vi "interface-doan.vi"() -> ()   [LabVIEW 2015]
panel:
  in  "?":T1(tab)
  out "Complete!":bool
  in  "?":bool
  in  "?":bool
  out "Process":dbl(knob) scale=0.0..100.0
  in  "?":path
  in  "GATE-3 3":i32(listbox)
  out "Complete!":bool
  in  "?":bool
  in  "?":bool
  out "Process":dbl(knob) scale=0.0..100.0
  in  "?":path
  in  "GATE-2 2":i32(listbox)
  out "Complete!":bool
  in  "?":bool
  in  "?":bool
  out "Process":dbl(knob) scale=0.0..100.0
  in  "?":path
  in  "GATE-1":i32(listbox)
  out "3":bool
  out "2":bool
  out "1":bool
  in  "Value 2":dbl
  in  "Value 1":dbl
  in  "Calibration":dbl
  in  "ERROR":errorcluster
  in  "ERROR":errorcluster
  out "Processing Chart":dbl(graph)
  out "WEIGHT PASS":bool
  out "Measurement\nValue":dbl
  out "Calculated\nValue":dbl
  out "Frame rate":dbl
  in  "DATA":string
  out "FOUND-QR":bool
  out "?":T2(plugin-control)
  # "GATE OUT"
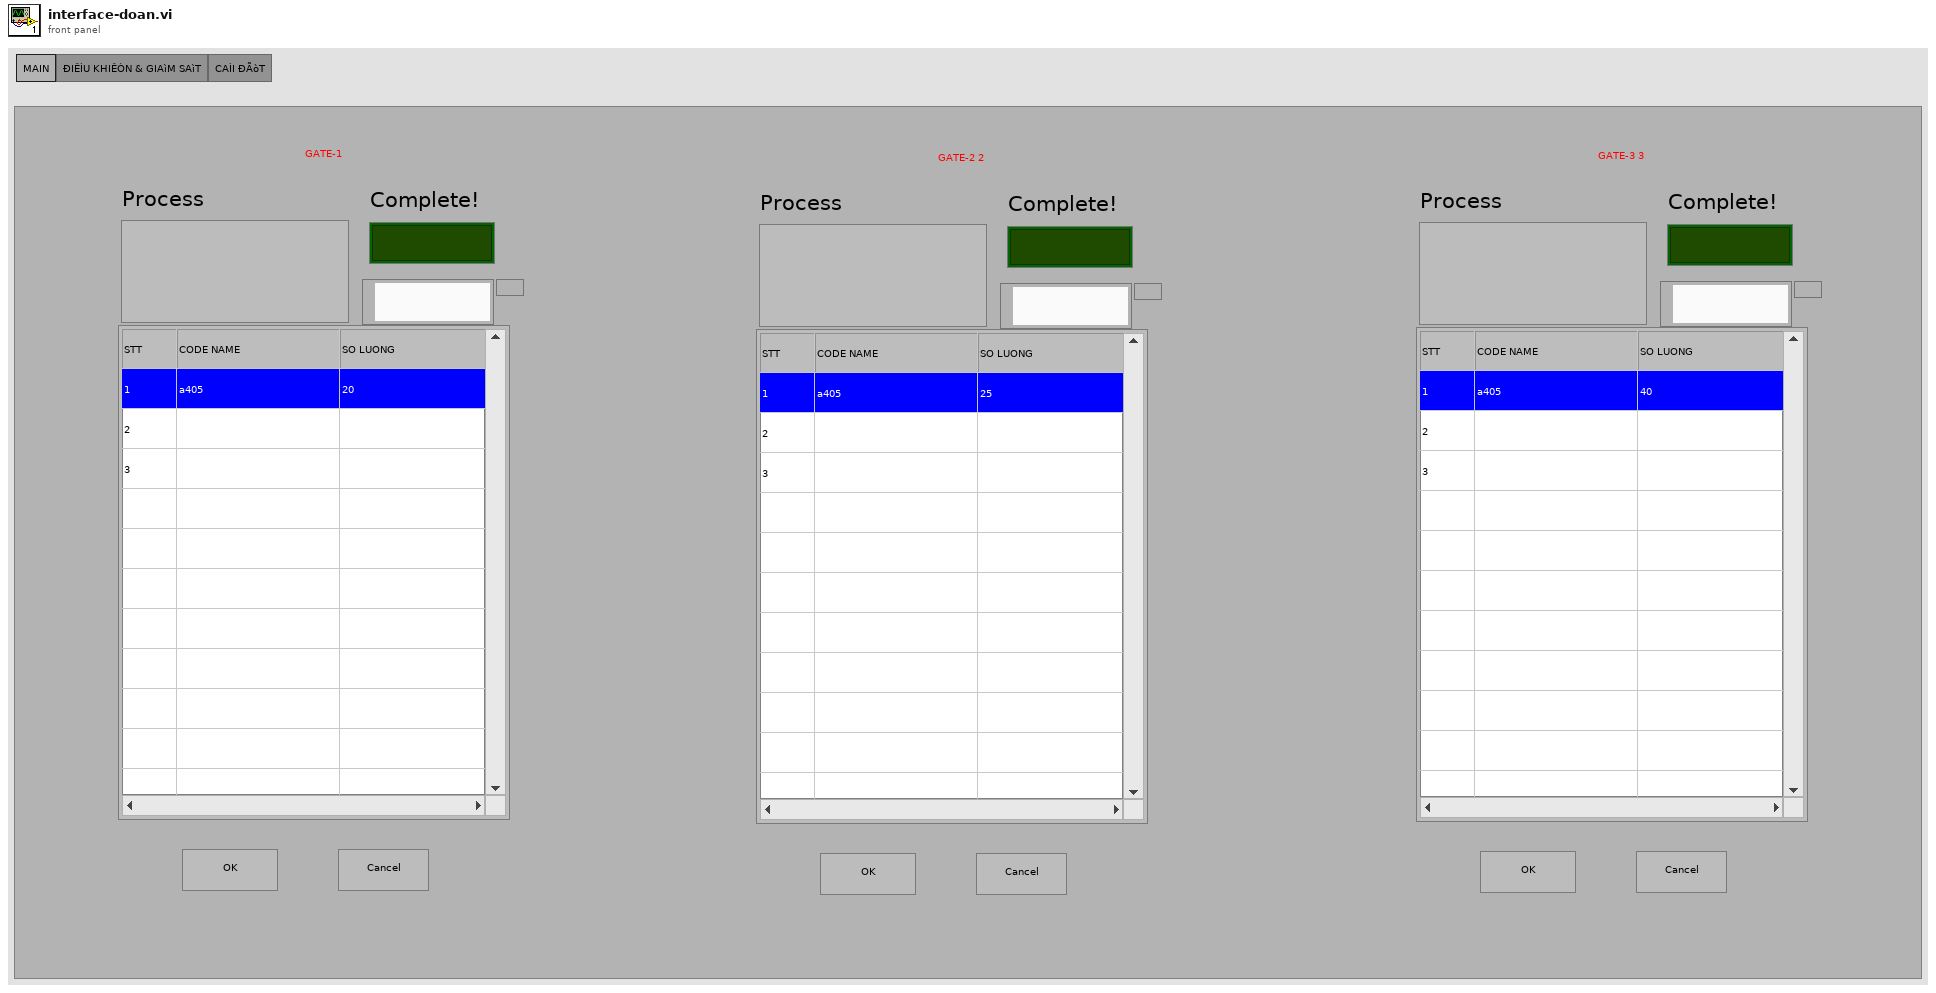
[diagram p1: front panel]
types:
  T1 = enum32{"MAIN", "ÐIÊÌU KHIÊÒN & GIAìM SAìT", "CAÌI ÐÃòT"}
  T2 = typedef "IMAQ Image.ctl" = refnum<image>
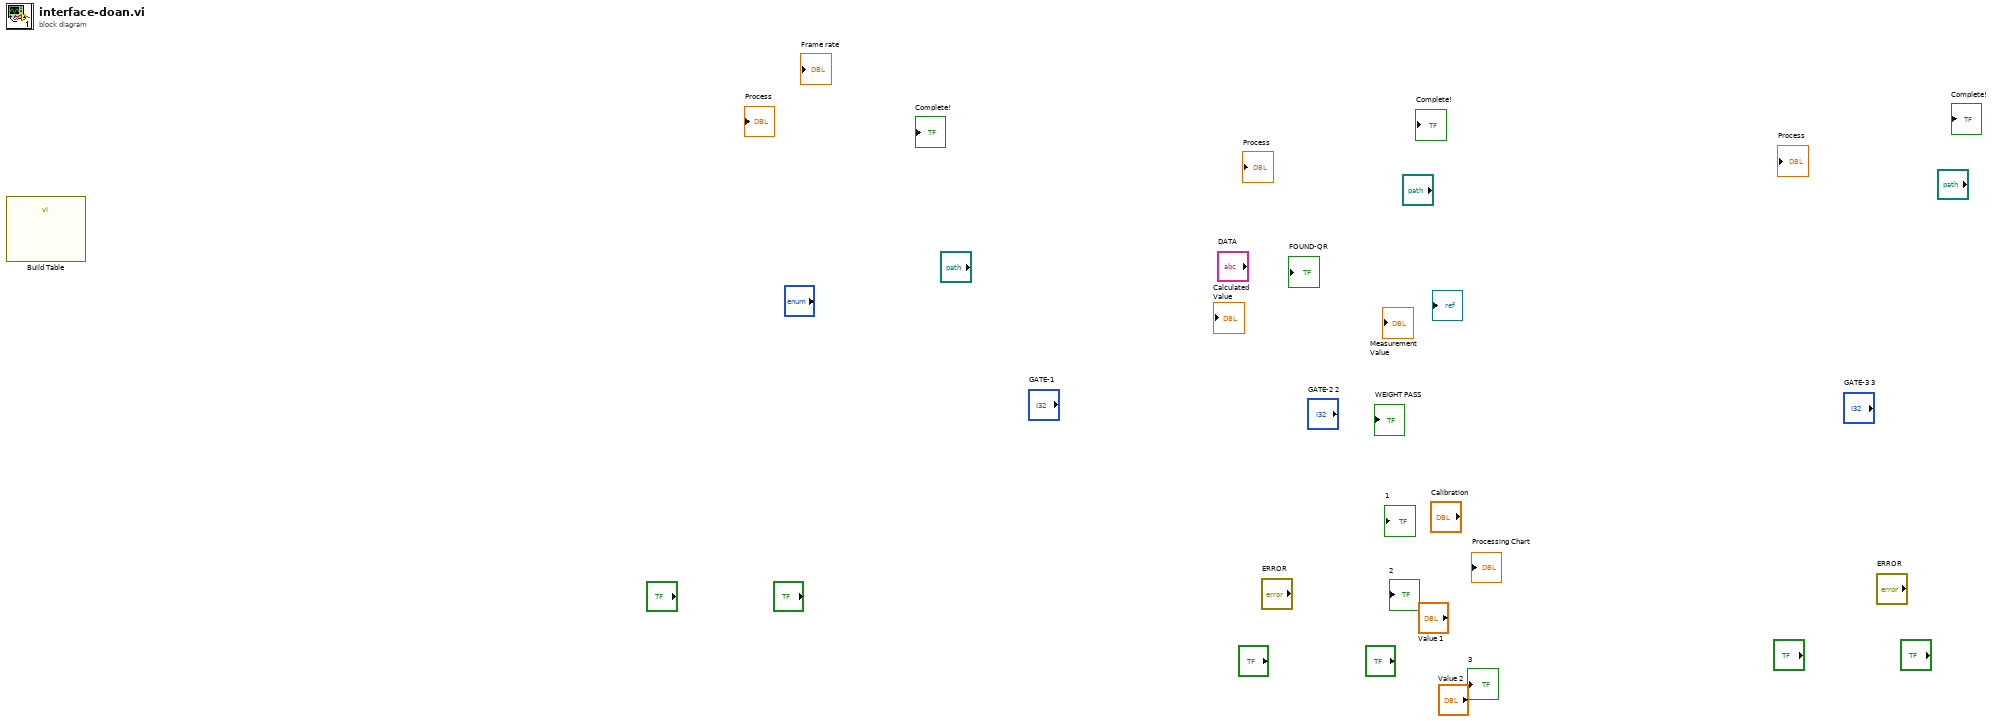
[diagram p0: block diagram]
diagram:
  n1 = call "Build Table"() -> ()  [unwired: 5 in, 7 out]
